vi "Init Global Arm Variables.vi"   [LabVIEW 2017]
uses:
  Global Arm Variables.vi
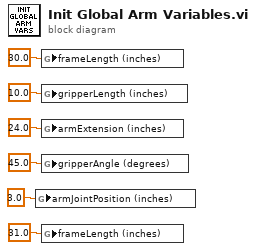
[diagram p0: block diagram]
diagram:
  n1 = global write "Global Arm Variables.vi" "armJointPosition (inches)"(3.0 ("armJointPosition")) -> ()
  n2 = global write "Global Arm Variables.vi" "frameLength (inches)"(30.0 ("arm Length")) -> ()
  n3 = global write "Global Arm Variables.vi" "gripperLength (inches)"(10.0 ("gripperLength")) -> ()
  n4 = global write "Global Arm Variables.vi" "armExtension (inches)"(24.0 ("armExtension")) -> ()
  n5 = global write "Global Arm Variables.vi" "gripperAngle (degrees)"(45.0 ("gripperAngle")) -> ()
  n6 = global write "Global Arm Variables.vi" "frameLength (inches)"(31.0 ("frameLength")) -> ()
